vi "Sixtypes Select.vi"() -> ()   [LabVIEW 2012]
doc: "This VI shows how you can read of different data types from a table named sixtypes in the LabVIEW.mdb database. \n\nThe table is created by the Sixtypes Insert VI, so it must be run before this VI in order to read data. Each of the values in the database table is a different data type and is converted by the Database Variant To Data function to their original LabVIEW data types."
uses:
  Connection.llb/DB Tools Open Connec (Path).vi
  NI_Database_API_64.lvlib
  _DB Variant To Data/Database Variant To Data.xnode
panel:
  out "Date/Time":string
  out "Binary (CDB)":cdb format="%.2f"
  out "Numeric (Double)":dbl format="%.7f"
  out "Numeric (Single)":sgl format="%.5f"
  out "Numeric (Long)":i32
  out "String":string
  # "Please refer to the VI Documentation (Ctrl-I) before running."
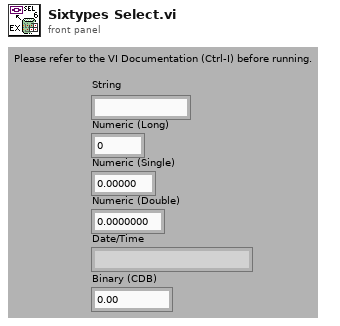
[diagram p1: front panel]
types:
  T1 = typedef "NI_Database_API_64.lvlib/Conn ObjectReference.ctl" = refnum<k1>
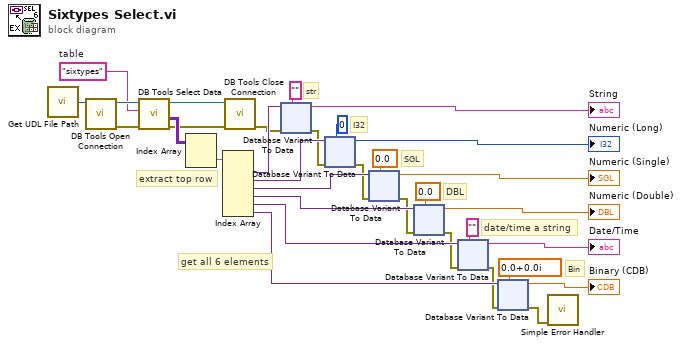
[diagram p0: block diagram]
diagram:
  w31 = "sixtypes"  # table
  # "get all 6 elements"
  # "extract top row"
  # "date/time a string"
  # "Bin"
  # "DBL"
  # "SGL"
  # "I32"
  # "str"
  n1 = call "Get UDL File Path.vi"() -> ("UDL file path"=w1:path)  [unwired: 1 in]
  n2 = call-poly "DB Tools Open Connection.vi"("connection information"=w1) -> ("error out"=w33:errorcluster, "connection reference"=w32:T1)  [unwired: 7 in]
  n3 = call "DB Tools Select Data.vi"("error in (no error)"=w33, "table"=w31, "connection reference"=w32) -> ("error out"=w4:errorcluster, "data"=w12:variant[][], "connection reference out"=w5:T1)  [unwired: 3 in]
  n4 = Index Array(array=w12) -> (element=w13:variant[])  [unwired: 2 in]
  n5 = Index Array(array=w13) -> (element #1=w30:variant, element #2=w29:variant, element #3=w28:variant, element #4=w27:variant, element #5=w26:variant, element #6=w25:variant)  [unwired: 6 in]
  n6 = call "DB Tools Close Connection.vi"("error in (no error)"=w4, "connection reference"=w5) -> ("error out"=w3:errorcluster)  [unwired: 5 in]
  n7 = xnode "Database Variant To Data"("database variant"=w30, "error in"=w3, "type"="" ("String")) -> ("data"=→"String":string, "error out"=w24:errorcluster)
  n8 = xnode "Database Variant To Data"("database variant"=w29, "error in"=w24, "type"=0 ("Numeric (Long)")) -> ("data"=→"Numeric (Long)":i32, "error out"=w23:errorcluster)
  n9 = xnode "Database Variant To Data"("database variant"=w28, "error in"=w23, "type"=sgl 0.0 ("Numeric (Single)")) -> ("data"=→"Numeric (Single)":sgl, "error out"=w22:errorcluster)
  n10 = xnode "Database Variant To Data"("database variant"=w27, "error in"=w22, "type"=0.0 ("Numeric (Double)")) -> ("data"=→"Numeric (Double)":dbl, "error out"=w21:errorcluster)
  n11 = xnode "Database Variant To Data"("database variant"=w26, "error in"=w21, "type"="" ("String")) -> ("data"=→"Date/Time":string, "error out"=w20:errorcluster)
  n12 = xnode "Database Variant To Data"("database variant"=w25, "error in"=w20, "type"=cdb 0.0+0.0i ("Binary (CDB)")) -> ("data"=→"Binary (CDB)":cdb, "error out"=w2:errorcluster)
  n13 = call <vilib>:"Simple Error Handler.vi"("error in (no error)"=w2) -> ()  [unwired: 4 in, 5 out]
